vi "EFW Get Property.vi"(8 "error in (no error)":errorcluster caption="错误输入（无错误）", 10 "pInfo":T1, 11 "ID":i32) -> (0 "error out":errorcluster caption="错误输出", 2 "pInfo out":T1, 3 "function return":u32(ring))   [LabVIEW 2012, in "EFW_filter.lvlib"]
doc: "EFW_API EFW_ERROR_CODE EFWGetProperty(int ID, EFW_INFO *pInfo);"
uses:
  <userlib>/EFW_filter/EFW_filter.lvlib
  <userlib>/EFW_filter/EFW_filter.dll
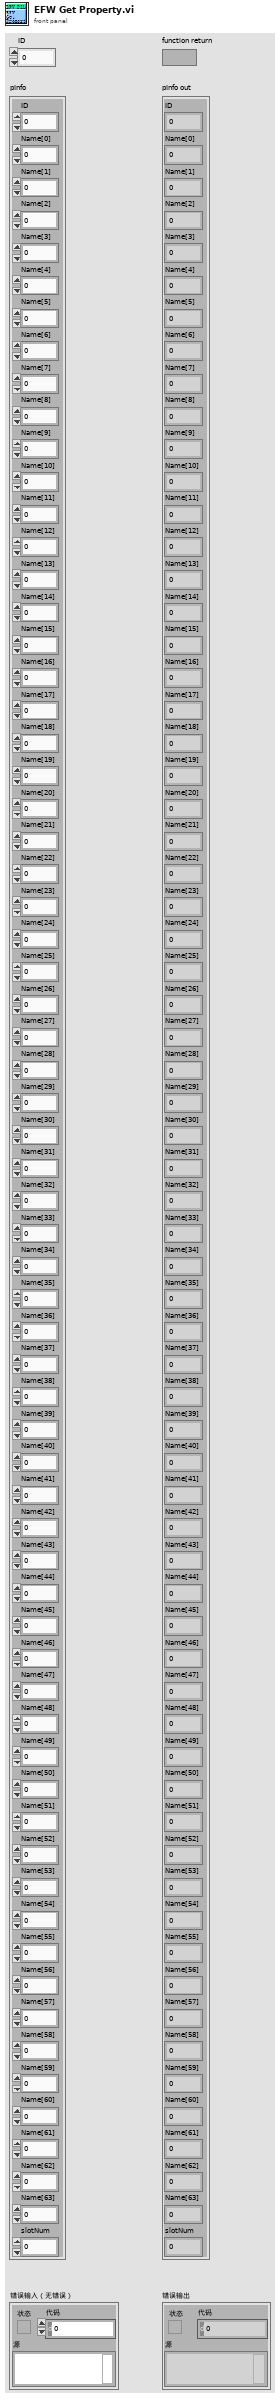
[diagram p1: front panel]
types:
  T1 = cluster{"ID":i32, "Name[0]":i8, "Name[1]":i8, "Name[2]":i8, "Name[3]":i8, "Name[4]":i8, "Name[5]":i8, "Name[6]":i8, "Name[7]":i8, "Name[8]":i8, "Name[9]":i8, "Name[10]":i8, "Name[11]":i8, "Name[12]":i8, "Name[13]":i8, "Name[14]":i8, "Name[15]":i8, "Name[16]":i8, "Name[17]":i8, "Name[18]":i8, "Name[19]":i8, "Name[20]":i8, "Name[21]":i8, "Name[22]":i8, "Name[23]":i8, "Name[24]":i8, "Name[25]":i8, "Name[26]":i8, "Name[27]":i8, "Name[28]":i8, "Name[29]":i8, "Name[30]":i8, "Name[31]":i8, "Name[32]":i8, "Name[33]":i8, "Name[34]":i8, "Name[35]":i8, "Name[36]":i8, "Name[37]":i8, "Name[38]":i8, "Name[39]":i8, "Name[40]":i8, "Name[41]":i8, "Name[42]":i8, "Name[43]":i8, "Name[44]":i8, "Name[45]":i8, "Name[46]":i8, "Name[47]":i8, "Name[48]":i8, "Name[49]":i8, "Name[50]":i8, "Name[51]":i8, "Name[52]":i8, "Name[53]":i8, "Name[54]":i8, "Name[55]":i8, "Name[56]":i8, "Name[57]":i8, "Name[58]":i8, "Name[59]":i8, "Name[60]":i8, "Name[61]":i8, "Name[62]":i8, "Name[63]":i8, "slotNum":i32}
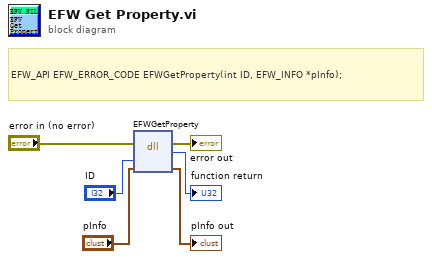
[diagram p0: block diagram]
diagram:
  # "EFW_API\tEFW_ERROR_CODE EFWGetProperty(int ID, EFW_INFO *pInfo);"
  n1 = dll-call lib="D:/Program Files (x86)/National Instruments/LabVIEW 2012/user.lib/EFW_filter/EFW_filter.*" fn="EFWGetProperty"(error in="error in (no error)", "ID"="ID", "pInfo"="pInfo") -> (error out=→"error out":errorcluster, →"function return":u32, "pInfo"=→"pInfo out":T1)  [unwired: 3 in, 1 out]
